vi "franch_OFDM_modulator.vi"(4 "error in (no error)":errorcluster, 5 "OFDM Parameters":T1={"FFT size (N)"=64, "Length of CP (Lc)"=8, "Null Tones"=[0, 30, 31, 32], "Number of OFDM Symbols (derived)"=1, "Training Sequence FFT size"=0, "Training Sequence Length of CP"=0}, 7 "input symbols":cdb[](array[numeric])) -> (0 "error out":errorcluster, 1 "OFDM Parameters out":T1={"FFT size (N)"=64, "Length of CP (Lc)"=8, "Null Tones"=[0, 30, 31, 32], "Number of OFDM Symbols (derived)"=1, "Training Sequence FFT size"=0, "Training Sequence Length of CP"=0}, 3 "output samples":cdb[](array[numeric]))   [LabVIEW 2012]
uses:
  OFDM_parameters.ctl
  <vilib>/Analysis/2dsp.llb/Inverse Complex FFT.vi
  <vilib>/Analysis/NI_AALPro.lvlib
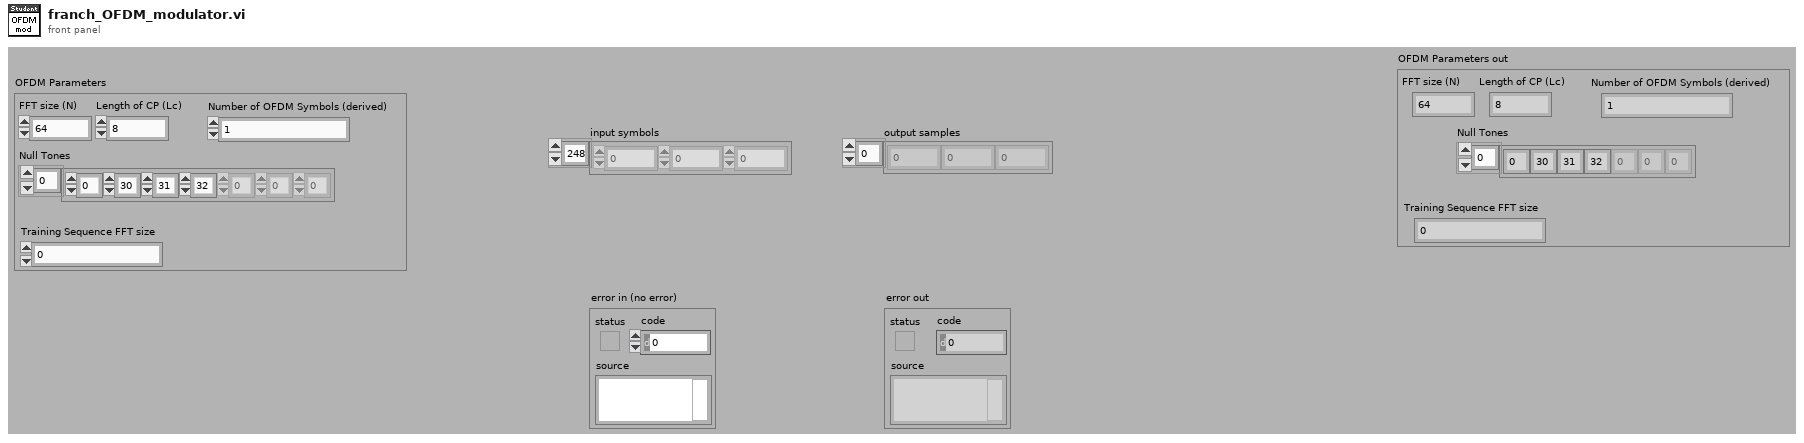
[diagram p1: front panel]
types:
  T1 = typedef "OFDM_parameters.ctl" = cluster{"FFT size (N)":i32, "Length of CP (Lc)":i32, "Null Tones":u32[], "Number of OFDM Symbols (derived)":i32, "Training Sequence FFT size":i32, "Training Sequence Length of CP":i32}
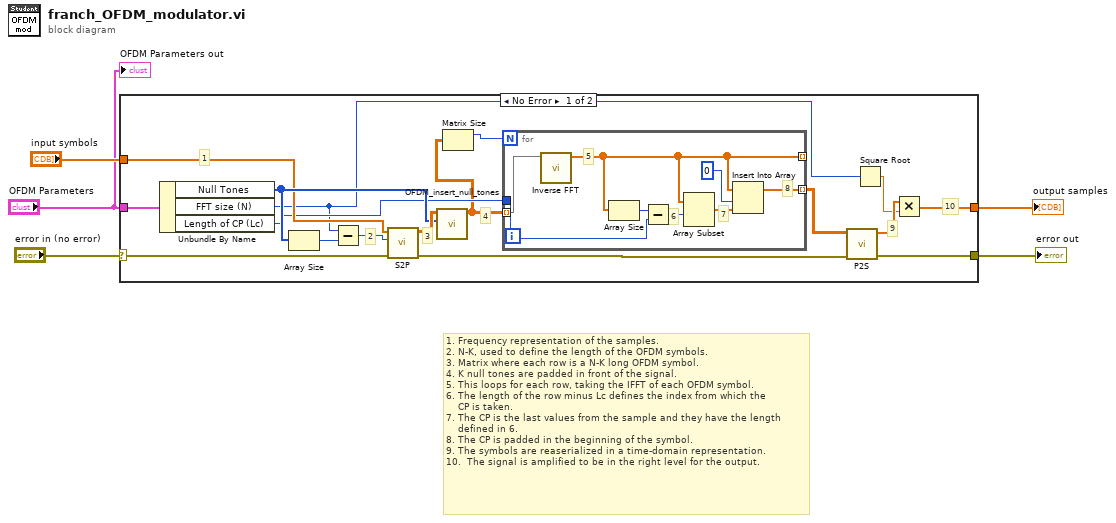
[diagram p0: block diagram]
diagram:
  # "1. Frequency representation of the samples.\n2. N-K, used to define the length of the OFDM symbols.\n3. Matrix where each row is a N-K long OFDM symbol.\n4. K null tones are padded in front of the signal.\n5. This loops for each row, taking the IFFT of each OFDM symbol.\n6. The length of the row minus Lc defines the index from which the \n    CP is taken.\n7. The CP is the last values from the sample and they have the length\n    defined in 6.\n8. The CP is padded in the beginning of the symbol.\n9. The symbols are reaserialized in a time-domain representation.\n10.  The signal is amplified to be in the right level for the output."
  n1 = case shown="No Error" "error in (no error)" {
    selector: "error in (no error)" -> [w14 w32]
    tunnel: "OFDM Parameters" -> [w22 _]
    tunnel: "input symbols" -> [w13 w31]
    tunnel: [w17 w32] -> w4
    tunnel: [w11 w31] -> w2
    frame No Error {
      # "10"
      # "9"
      # "4"
      # "3"
      # "2"
      # "1"
      n2 = Unbundle By Name(w22) -> ("Null Tones"=w16:u32[], "FFT size (N)"=w9:i32, "Length of CP (Lc)"=w10:i32)
      n3 = Array Size(array=w16) -> (size(s)=w15:i32)
      n4 = Subtract(x=w9, y=w15) -> (x-y=w21:i32)
      n5 = call "S2P.vi"("error in (no error)"=w14, "block size"=w21, "serial input"=w13) -> ("error out"=w18:errorcluster, "parallel output"=w20:cdb[][])  [unwired: 3 in]
      n6 = call "OFDM_insert_null_tones.vi"("null tones"=w16, "input"=w20) -> ("output"=w7:cdb[][])  [unwired: 5 in]
      n7 = Matrix Size(0:w7) -> (1:w6:i32)  [unwired: 1 out]
      n8 = for {
        N: w6 -> [_]
        tunnel: w7 -> [w26] mode=indexing
        tunnel: [w24] -> w19 mode=indexing
        tunnel: [w25] -> _ mode=indexing
        tunnel: w10 -> [w23]
        # "8"
        # "7"
        # "6"
        # "5"
        n9 = call-poly <vilib>:"Inverse FFT.vi"("FFT {X}"=w26) -> ("X"=w25:cdb[])  [unwired: 9 in, 1 out]
        n10 = Array Size(array=w25) -> (size(s)=w30:i32)
        n11 = Subtract(x=w30, y=w23) -> (x-y=w29:i32)
        n12 = Array Subset(array=w25, index=w29) -> (w28:cdb[])  [unwired: 1 in]
        n13 = Insert Into Array(array=w25, index=0, new element=w28) -> (w24:cdb[])
      }
      n14 = call "P2S.vi"("error in (no error)"=w18, "parallel input"=w19) -> ("error out"=w17:errorcluster, "serial output"=w12:cdb[])  [unwired: 3 in, 1 out]
      n15 = Square Root(x=w9) -> (sqrt(x)=w8:dbl)
      n16 = Multiply(x=w12, y=w8) -> (x*y=w11:cdb[])
    }
    frame Error {
    }
  }
  "error out" <- w4
  "output samples" <- w2
  "OFDM Parameters out" <- "OFDM Parameters"
